vi "Name Value Metadata Interface.vi"(0 "Save Path":path, 7 "Input Tags Path":path) -> ()   [LabVIEW 2020]
uses:
  <vilib>/Utility/miscctls.llb/LVPointTypeDef.ctl
  Name Value Controls/Name Value Data Type Def.ctl
  <vilib>/Utility/file.llb/Read Delimited Spreadsheet (string).vi
panel:
  in  "Group Name Input":string
  in  "Tag Group 0":bool
  in  "Tag Group 6":bool
  in  "Tag Group 5":bool
  in  "Tag Group 4":bool
  in  "Tag Group 3":bool
  in  "Tag Group 2":bool
  in  "Tag Group 1":bool
  in  "Cancel":bool
  in  "Save":bool
  in  "Notes":string
  in  "Update Preset":bool
  in  "Save Preset":bool
  in  "Preset":u16(ring) items=["None", "Testing Two", "Testing"]
  in  "Clear All Tags":bool
  in  "Clear Tags":bool
  in  "Remove Group":bool
  in  "Add Group":bool
  in  "Metadata Tags":string[][](array[string])
  # "Name"
  # "Value"
  # "Value"
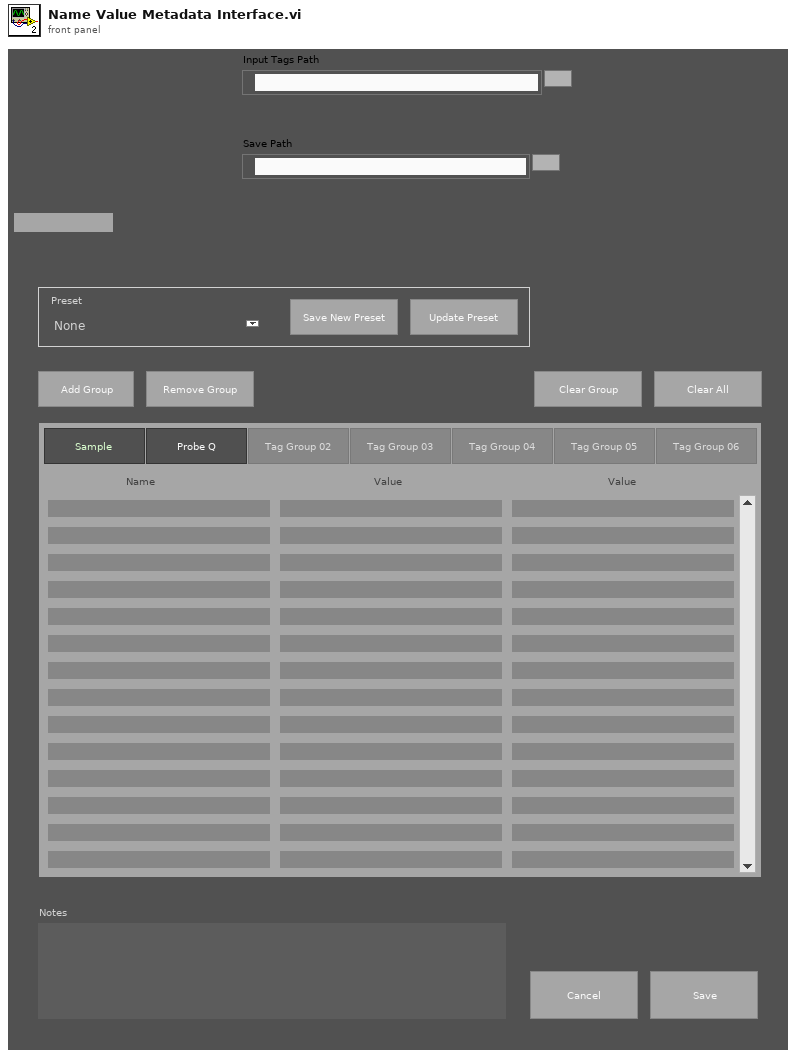
[diagram p1: front panel]
types:
  T1 = enum16{"Always On", "Always Off", "Off While Running"}
  T2 = typedef "LVPointTypeDef.ctl" = cluster{"Horizontal":i16, "Vertical":i16}
  T3 = enum8{"Enabled", "Disabled", "Disabled and Grayed Out"}
  T4 = typedef "Name Value Data Type Def.ctl" = cluster{"Sorted Tags":string[], "First Letters":string[], "Letter Indices":i32[]}
  T5 = typedef "LVBoundsTypeDef.ctl" = cluster{"Width":u32, "Height":u32}
  T6 = typedef "LVRectTypeDef.ctl" = cluster{"Left":i16, "Top":i16, "Right":i16, "Bottom":i16}
  T7 = enum32{"Invalid", "Standard", "Closed", "Hidden", "Minimized", "Maximized"}
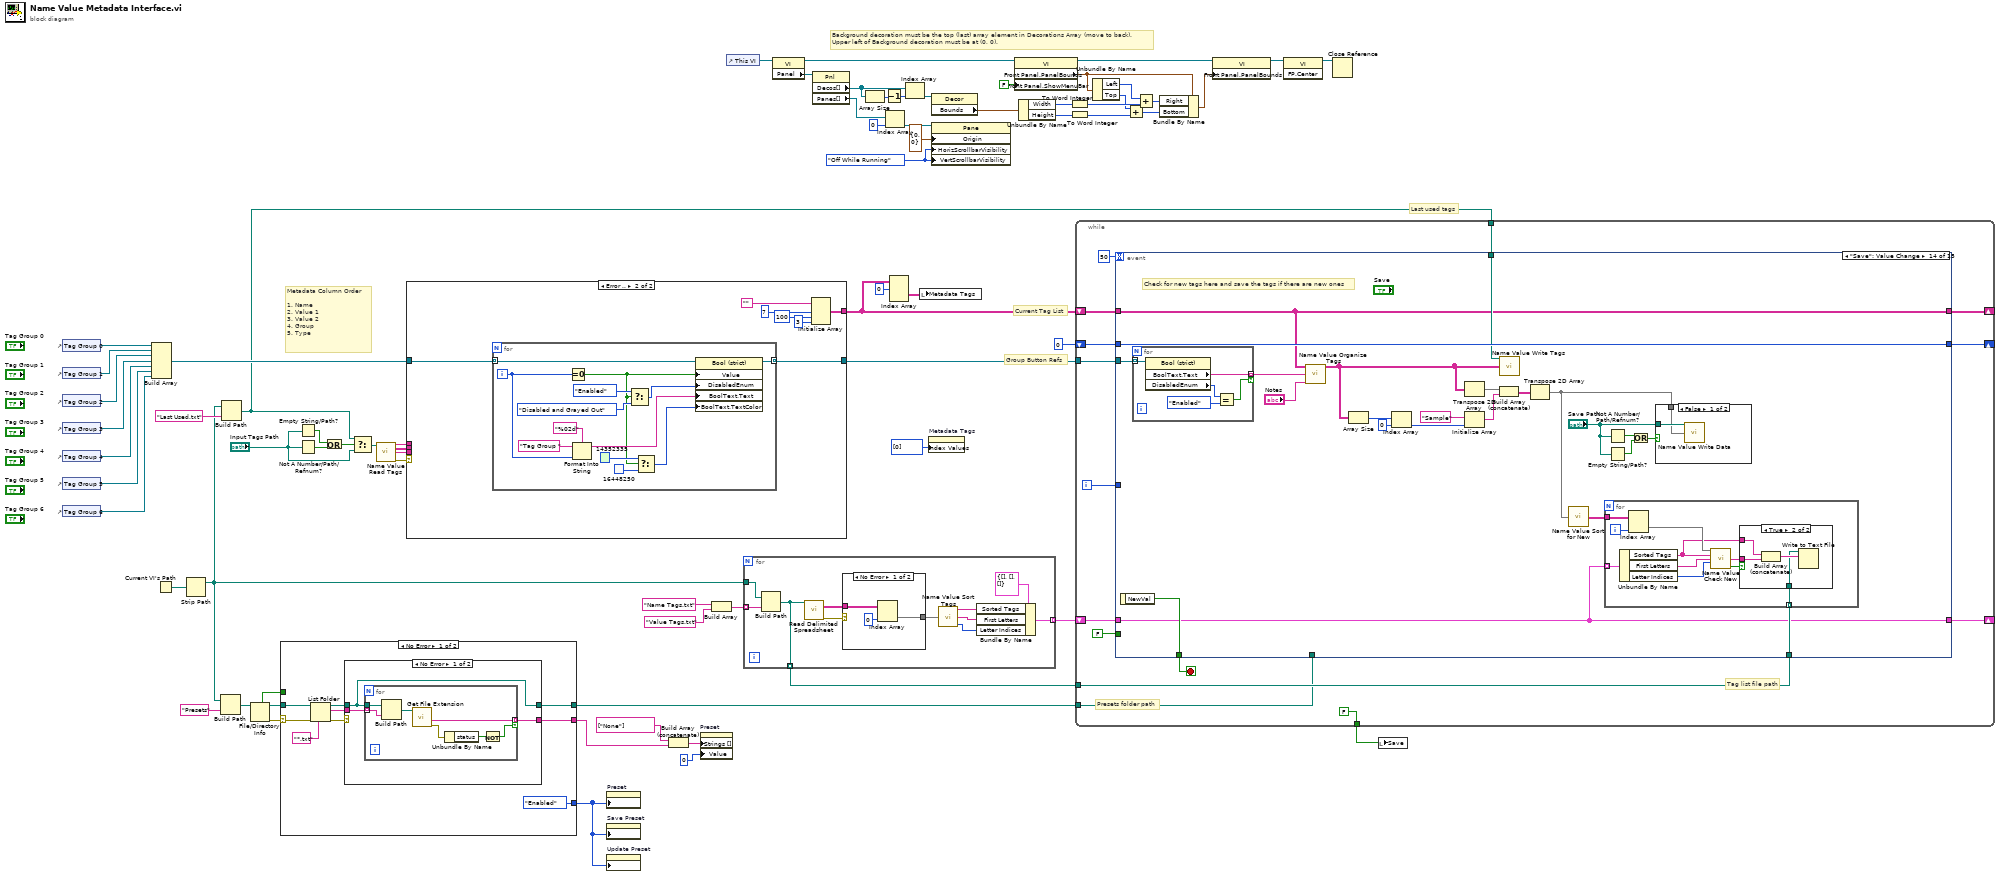
[diagram p0: block diagram]
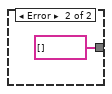
[diagram p2: hidden frame]
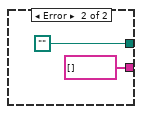
[diagram p3: hidden frame]
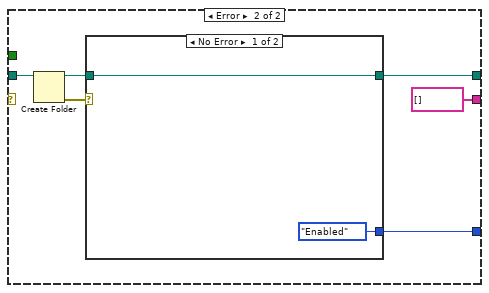
[diagram p4: hidden frame]
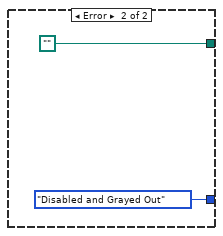
[diagram p5: hidden frame]
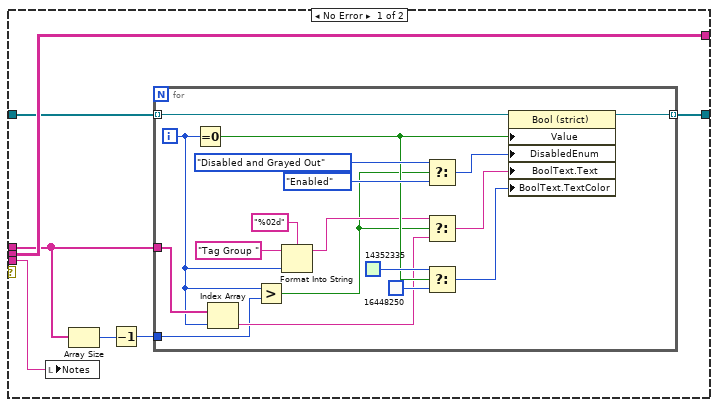
[diagram p6: hidden frame]
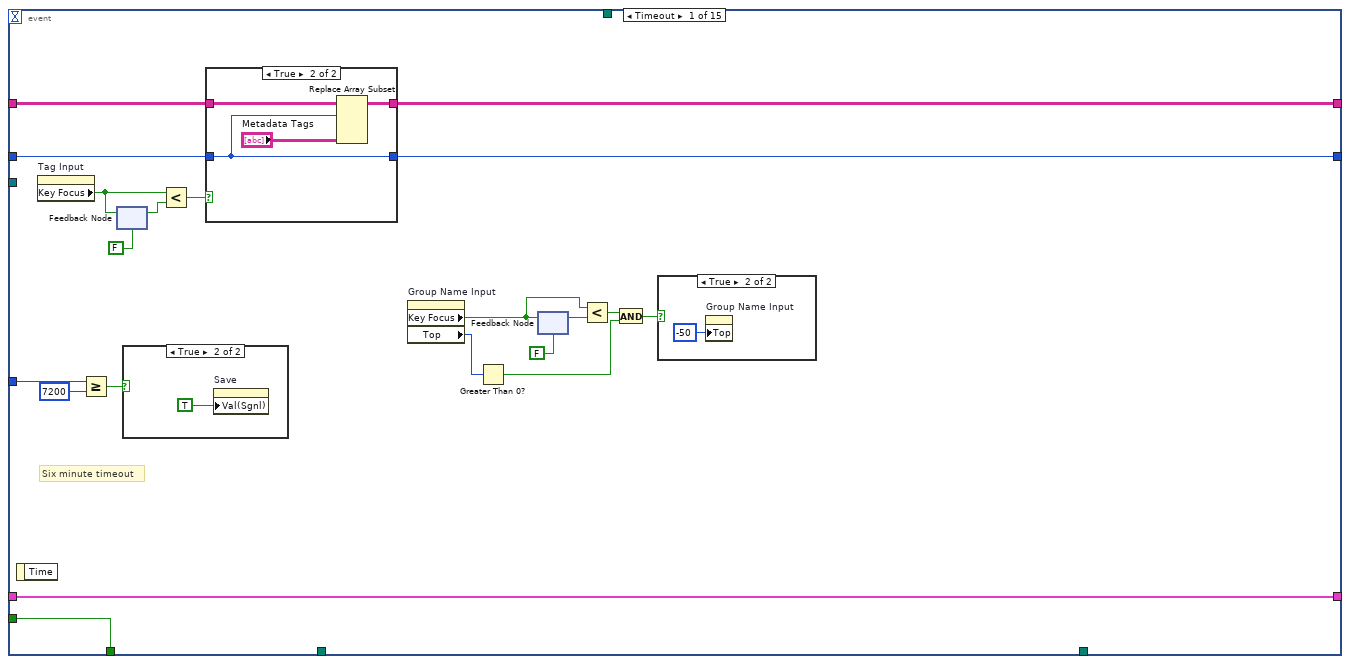
[diagram p7: hidden frame]
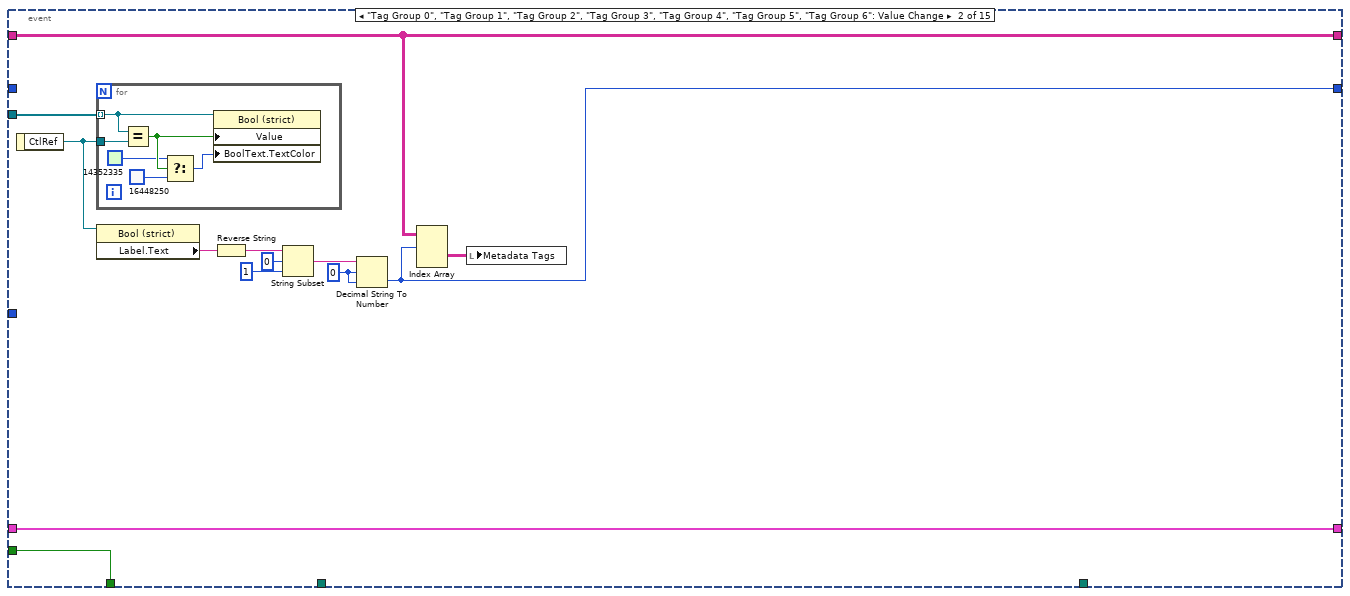
[diagram p11: hidden frame]
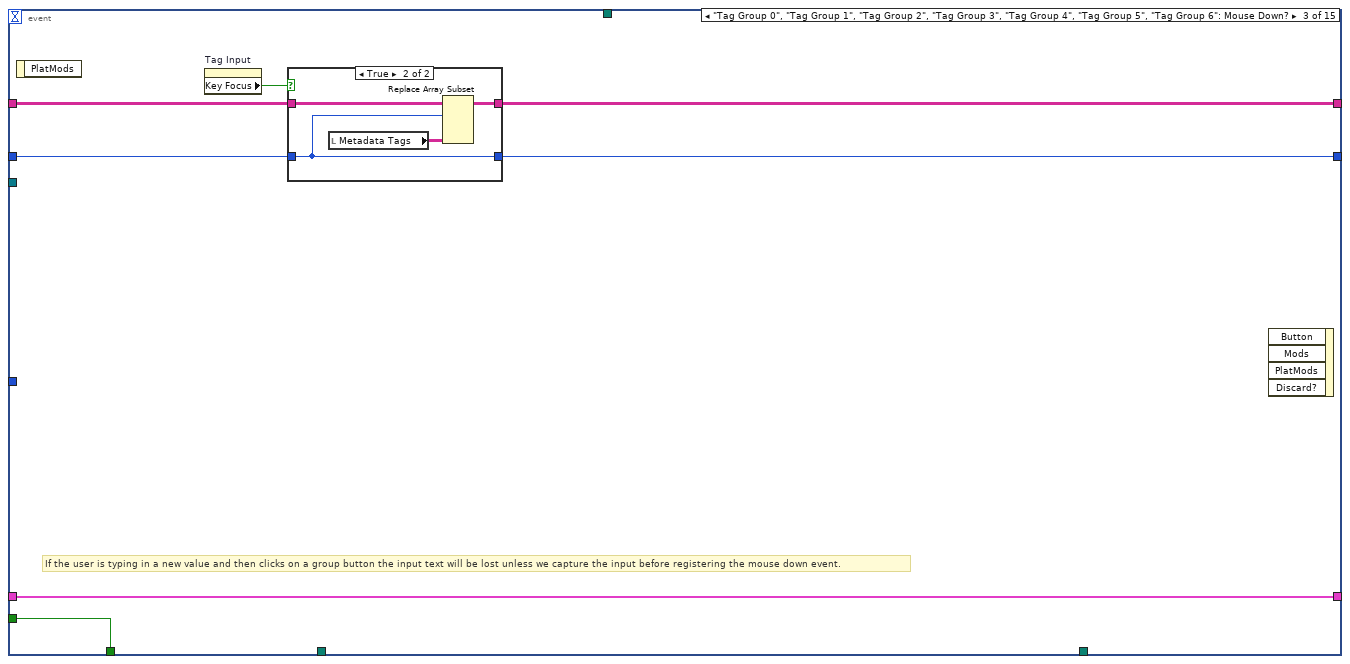
[diagram p12: hidden frame]
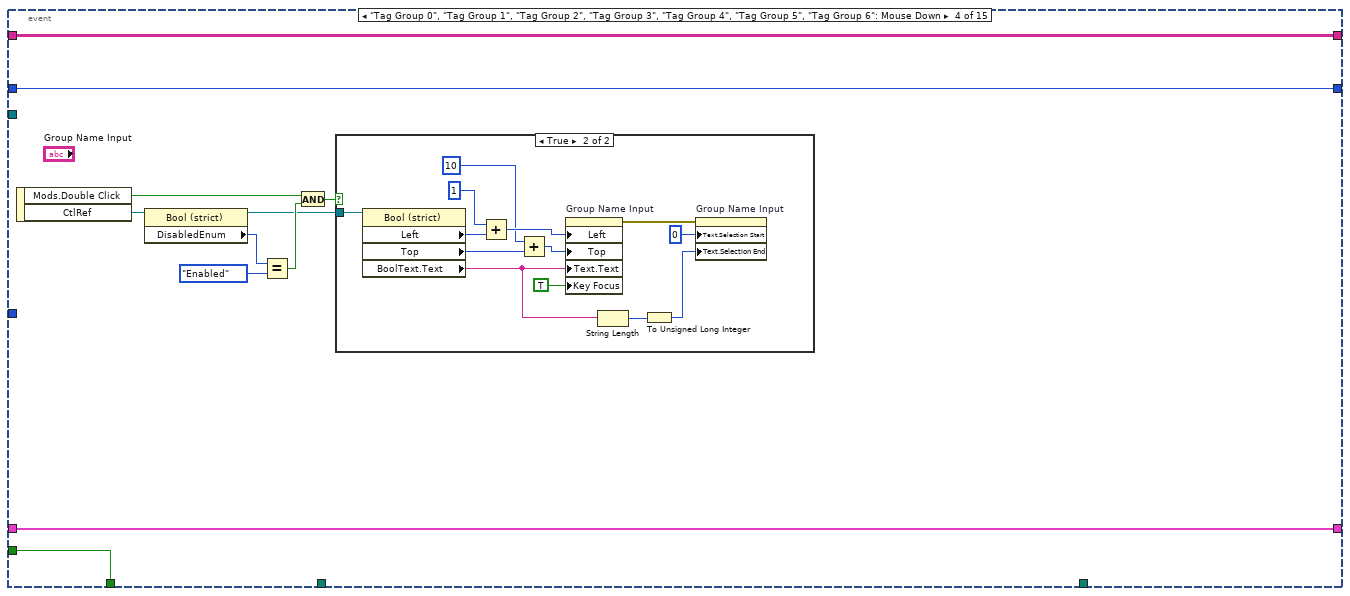
[diagram p14: hidden frame]
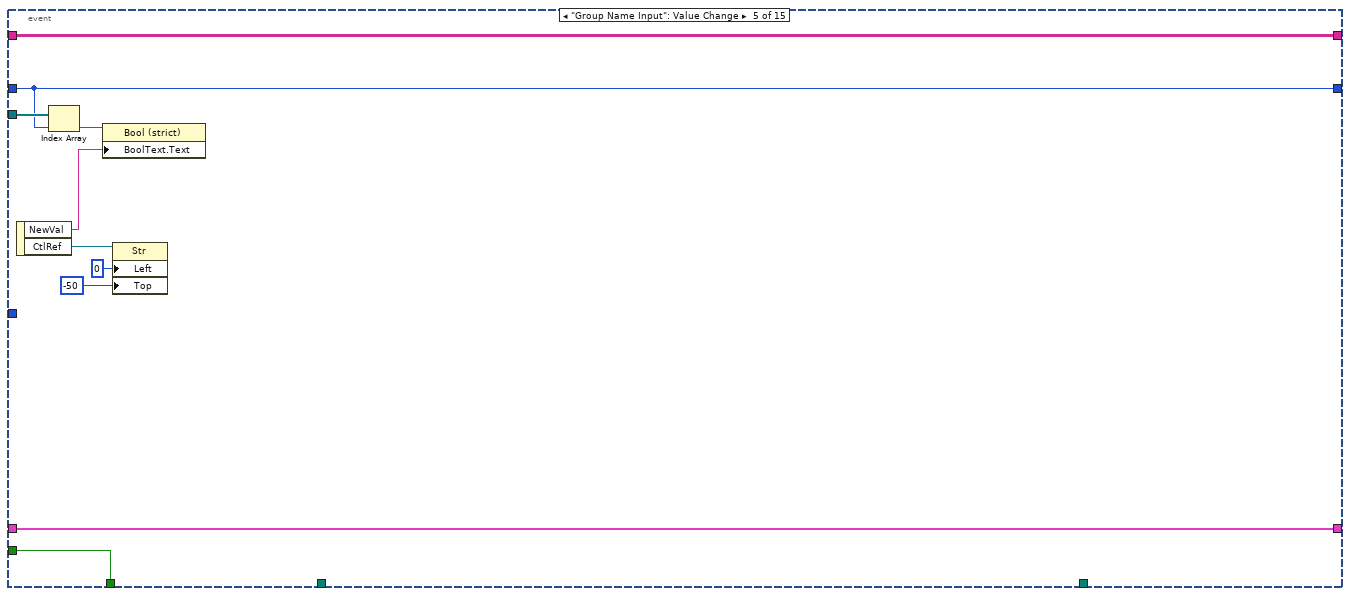
[diagram p16: hidden frame]
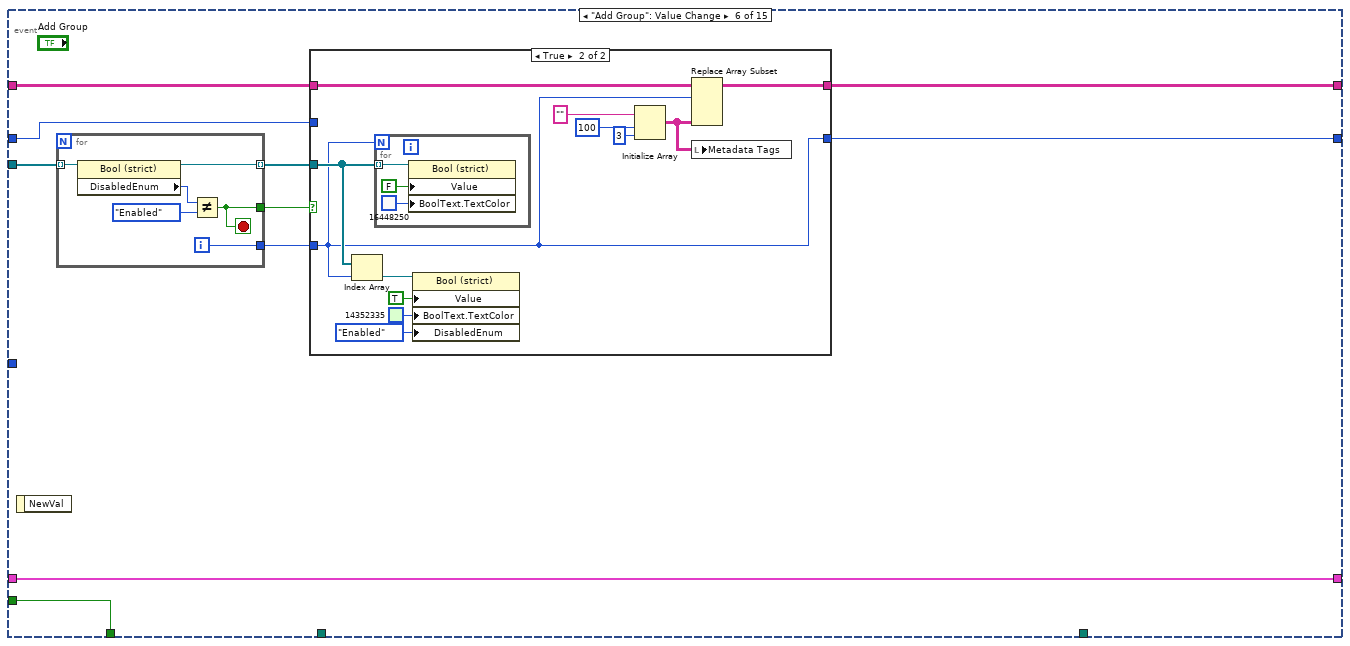
[diagram p17: hidden frame]
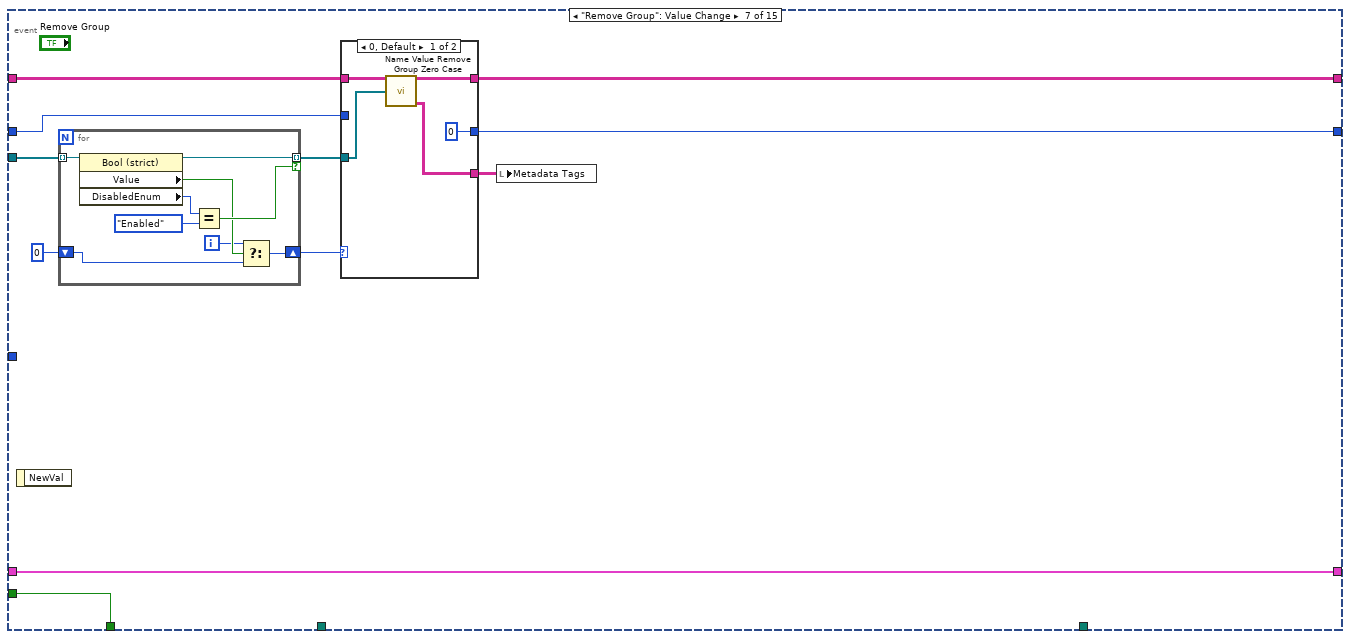
[diagram p19: hidden frame]
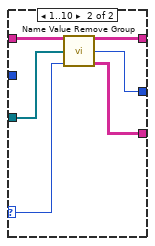
[diagram p20: hidden frame]
diagram:
  w62 = T1."Off While Running" ("Vertical Scrollbar Visibility")
  # "Last used tags"
  # "Group Button Refs"
  # "Metadata Column Order\n\n1. Name\n2. Value 1\n3. Value 2\n4. Group\n5. Type"
  # "Current Tag List"
  # "Background decoration must be the top (last) array element in Decorations Array (move to back).\nUpper left of Background decoration must be at (0, 0)."
  n1 = control-ref of="Tag Group 0"() -> (w46:refnum<vi>)
  n2 = control-ref of="Tag Group 1"() -> (w45:refnum<vi>)
  n3 = control-ref of="Tag Group 2"() -> (w44:refnum<vi>)
  n4 = control-ref of="Tag Group 3"() -> (w43:refnum<vi>)
  n5 = control-ref of="Tag Group 4"() -> (w42:refnum<vi>)
  n6 = control-ref of="Tag Group 5"() -> (w41:refnum<vi>)
  n7 = control-ref of="Tag Group 6"() -> (w40:refnum<vi>)
  n8 = Build Array(w46, w45, w44, w43, w42, w41, w40) -> (w38:refnum<vi>[])
  n9 = Current VI's Path() -> (path=w49:path)
  n10 = Strip Path(path=w49) -> (stripped path=w4:path)  [unwired: 1 out]
  n11 = Build Path(base path=w4, name or relative path="Presets") -> (appended path=w30:path)
  n12 = Build Path(base path=w4, name or relative path="Last Used.txt") -> (appended path=w15:path)
  n13 = File/Directory Info(path=w30) -> (path out=w27:path, directory=w28:bool, error out=w29:errorcluster)  [unwired: 1 in, 4 out]
  n14 = case shown="No Error" w29 {
    selector: w29 -> [w79 _]
    tunnel: w28 -> [_ _]
    tunnel: w27 -> [w80 w98]
    tunnel: [w73 w95] -> w22
    tunnel: [w75 string[] []] -> w24
    tunnel: [T3."Enabled" ("Disabled") w93] -> w21
    frame No Error {
      n15 = List Folder(path=w80, pattern="*.txt", error in=w79) -> (path out=w76:path, filenames=w77:string[], error out=w74:errorcluster)  [unwired: 1 in, 1 out]
      n16 = case shown="No Error" w74 {
        tunnel: w77 -> [w83 _]
        tunnel: w76 -> [w81 _]
        tunnel: [w82 string[] []] -> w75
        tunnel: [w81 path ""] -> w73
        frame No Error {
          n17 = for {
            tunnel: w83 -> [w89] mode=indexing
            tunnel: w81 -> [w90]
            tunnel: [w87] -> w82 mode=indexing if=w84
            n18 = Build Path(base path=w90, name or relative path=w89) -> (appended path=w88:path)
            n19 = call <vilib>:"Get File Extension.vi"("file"=w88) -> ("error out"=w86:errorcluster, "filename without extension"=w87:string)  [unwired: 6 in, 3 out]
            n20 = Unbundle By Name(w86) -> ("status"=w85:bool)
            n21 = Not(x=w85) -> (.not. x?=w84:bool)
          }
        }
        frame Error {
        }
      }
    }
    frame Error {
      n22 = Create Folder(path (use dialog)=w98) -> (created path=w96:path, error out=w97:errorcluster)  [unwired: 2 in, 1 out]
      n23 = case shown="No Error" w97 {
        tunnel: w96 -> [w100 _]
        tunnel: [w100 path ""] -> w95
        tunnel: [T3."Enabled" ("Disabled") T3."Disabled and Grayed Out" ("Disabled")] -> w93
        frame No Error {
        }
        frame Error {
        }
      }
    }
  }
  n24 = Empty String/Path?(string/path="Input Tags Path") -> (empty?=w19:bool)
  n25 = Not A Number/Path/Refnum?(number/path/refnum="Input Tags Path") -> (NaN/Path/Refnum?=w18:bool)
  n26 = Or(x=w19, y=w18) -> (x .or. y?=w17:bool)
  n27 = Select(t=w15, s=w17, f="Input Tags Path") -> (s? t:f=w20:path)
  n28 = call "Name Value Read Tags.vi"("Path"=w20) -> ("Group Names"=w34:string[], "Tags"=w33:string[][][], "Notes"=w32:string, "Error Out"=w35:errorcluster)  [unwired: 11 in]
  n29 = case shown="Error .." w35 {
    tunnel: w38 -> [w108 w134]
    tunnel: [w107 w133] -> w37
    tunnel: [w109 w130] -> w10
    tunnel: w34 -> [w106 _]
    tunnel: w33 -> [w109 _]
    tunnel: w32 -> [w103 _]
    frame No Error {
      n30 = local write "Notes"(w103) -> ()
      n31 = Array Size(array=w106) -> (size(s)=w105:i32)
      n32 = Decrement(x=w105) -> (x-1=w104:i32)
      n33 = for {
        tunnel: w108 -> [w127] mode=indexing
        tunnel: [w126] -> w107 mode=indexing
        tunnel: w106 -> [w114]
        tunnel: w104 -> [w110]
        i -> [w112]
        n34 = Equal To 0?(x=w112) -> (x = 0?=w117:bool)
        n35 = Index Array(array=w114, index=w112) -> (element=w113:string)
        n36 = Greater?(x=w112, y=w110) -> (0:w111:bool)
        n37 = Format Into String(format string="%02d", initial string="Tag Group ", w112) -> (resulting string=w116:string)  [unwired: 1 in, 1 out]
        n38 = Select(t=T3."Disabled and Grayed Out" ("Disabled"), s=w111, f=T3."Enabled" ("Disabled")) -> (s? t:f=w124:T3)
        n39 = Select(t=w116, s=w111, f=w113) -> (s? t:f=w115:string)
        n40 = Select(t=u32 14352335 ("Color Box"), s=w117, f=u32 16448250) -> (s? t:f=w118:u32)
        n41 = property class="Bool (strict)"(reference=w127, "Value"=w117, "DisabledEnum"=w124, "BoolText.Text"=w115, "BoolText.TextColor"=w118) -> (reference out=w126:refnum<vi>)  [unwired: 1 in, 1 out]
      }
    }
    frame Error {
      n42 = for {
        tunnel: w134 -> [w147] mode=indexing
        tunnel: [w146] -> w133 mode=indexing
        i -> [w140]
        n43 = Equal To 0?(x=w140) -> (x = 0?=w135:bool)
        n44 = Format Into String(format string="%02d", initial string="Tag Group ", w140) -> (resulting string=w139:string)  [unwired: 1 in, 1 out]
        n45 = Select(t=T3."Enabled" ("Disabled"), s=w135, f=T3."Disabled and Grayed Out" ("Disabled")) -> (s? t:f=w144:T3)
        n46 = Select(t=u32 14352335 ("Color Box"), s=w135, f=u32 16448250) -> (s? t:f=w136:u32)
        n47 = property class="Bool (strict)"(reference=w147, "Value"=w135, "DisabledEnum"=w144, "BoolText.Text"=w139, "BoolText.TextColor"=w136) -> (reference out=w146:refnum<vi>)  [unwired: 1 in, 1 out]
      }
      n48 = Initialize Array("", 7 ("dimension size"), 100 ("dimension size"), 3 ("dimension size")) -> (w130:string[][][])
    }
  }
  n49 = property on="Preset" class="Ring (strict)"("DisabledEnum"=w21) -> ()  [unwired: 2 in, 2 out]
  n50 = property on="Save Preset" class="Bool"("DisabledEnum"=w21) -> ()  [unwired: 2 in, 2 out]
  n51 = property on="Update Preset" class="Bool"("DisabledEnum"=w21) -> ()  [unwired: 2 in, 2 out]
  n52 = Build Array (concatenate)(string[] ["None"] ("Strings []"), w24) -> (w25:string[])
  n53 = property on="Preset" class="Ring (strict)"("Strings []"=w25, "Value"=u16 0) -> ()  [unwired: 2 in, 2 out]
  n54 = Build Array("Name Tags.txt", "Value Tags.txt") -> (w5:string[])
  n55 = control-ref of="This VI"() -> (w14:refnum<vi>)
  n56 = for {
    tunnel: [w151] -> w3 mode=indexing
    tunnel: w5 -> [w150] mode=indexing
    tunnel: w4 -> [w149]
    tunnel: [w148] -> w2 mode=indexing
    n57 = Build Path(base path=w149, name or relative path=w150) -> (appended path=w148:path)
    n58 = call-poly <vilib>:"Read Delimited Spreadsheet.vi"("file path (dialog if empty)"=w148) -> ("all rows"=w158:string[][], "error out"=w157:errorcluster)  [unwired: 9 in, 4 out]
    n59 = case shown="No Error" w157 {
      tunnel: w158 -> [w161 _]
      tunnel: [w159 string[] [] ("all rows")] -> w156
      frame No Error {
        n60 = Index Array(array=w161, index (col)=0 ("disabled index (col)")) -> (element=w159:string[])  [unwired: 1 in]
      }
      frame Error {
      }
    }
    n61 = call "Name Value Sort Tags.vi"("Tags"=w156) -> ("Sorted Tags"=w154:string[], "First Letters"=w153:string[], "Letter Indices"=w152:i32[])  [unwired: 12 in]
    n62 = Bundle By Name(cluster=T4 {"Sorted Tags"=[], "First Letters"=[], "Letter Indices"=[]} ("Tag Data"), "Sorted Tags"=w154, "First Letters"=w153, "Letter Indices"=w152) -> (w151:T4)
  }
  n63 = property class="VI"(reference=w14) -> (reference out=w63:refnum<vi>, "Panel"=w56:refnum<vi>)  [unwired: 1 in, 1 out]
  n64 = property class="Pnl"(reference=w56) -> ("Decos[]"=w48:refnum<vi>[], "Panes[]"=w59:refnum<vi>[])  [unwired: 1 in, 2 out]
  n65 = Array Size(array=w48) -> (size(s)=w55:i32)
  n66 = Decrement(x=w55) -> (x-1=w47:i32)
  n67 = Index Array(array=w59, index=0) -> (element=w58:refnum<vi>)
  n68 = Index Array(array=w10, index (dim 0)=0 ("index (page)")) -> (element=w8:string[][])  [unwired: 2 in]
  n69 = Index Array(array=w48, index=w47) -> (element=w61:refnum<vi>)
  n70 = local write "Metadata Tags"(w8) -> ()
  n71 = property on="Metadata Tags" class="Arr (strict)"("Index Values"=u32[] [0]) -> ()  [unwired: 2 in, 2 out]
  n72 = property class="Decor"(reference=w61) -> ("Bounds"=w64:T5)  [unwired: 1 in, 2 out]
  n73 = property class="Pane"(reference=w58, "Origin"=T2 {"Horizontal"=0, "Vertical"=0}, "HorizScrollbarVisibility"=w62, "VertScrollbarVisibility"=w62) -> ()  [unwired: 1 in, 2 out]
  n74 = property class="VI"(reference=w63, "Front Panel.ShowMenuBar"=FALSE ("Front Panel Window:Show Menu Bar")) -> (reference out=w65:refnum<vi>, "Front Panel.PanelBounds"=w66:T6)  [unwired: 1 in, 1 out]
  n75 = Unbundle By Name(w64) -> ("Width"=w69:u32, "Height"=w71:u32)
  n76 = To Word Integer(number=w69) -> (16bit integer=w70:i16)
  n77 = To Word Integer(number=w71) -> (16bit integer=w51:i16)
  n78 = while {
    tunnel: w37 -> [w175]
    shift-right: [w168] -> _
    shift-left: w10 -> [w174]
    shift-right: [w172] -> _
    shift-left: 0 -> [w173]
    tunnel: w2 -> [w170]
    tunnel: w15 -> [w169]
    tunnel: w22 -> [w167]
    shift-right: [w164] -> _
    shift-left: w3 -> [w165]
    tunnel: [FALSE] -> w1
    i -> [w166]
    stop <- w176 stop-if-true
    # "Presets folder path"
    # "Tag list file path"
    n79 = event shown="[13] \"Save\": Value Change" {
      selector: _ -> [_ _ _ _ _ _ _ _ _ _ _ _ _ _ _]
      dyn-events: _ -> [_ _ _ _ _ _ _ _ _ _ _ _ _ _ _]
      timeout: 50 -> [_ _ _ _ _ _ _ _ _ _ _ _ _ _ _]
      tunnel: FALSE -> [w197 w218 w231 w248 w271 w281 w315 w363 w389 w399 w419 w465 w491 _ _]
      tunnel: [w197 w218 w231 w248 w271 w281 w315 w363 w389 w399 w419 w465 w491 w532 TRUE ("NewVal")] -> w176
      tunnel: w175 -> [_ w217 _ _ w266 w273 w314 _ _ _ w409 w463 w489 w530 _]
      tunnel: [w190 w208 w229 w247 w270 w275 w310 w351 w385 w392 w402 w450 w480 w523 w556] -> w168
      tunnel: w174 -> [w192 w208 w230 w247 w270 w276 w311 w351 w386 _ w405 w450 w480 w523 w556]
      tunnel: w173 -> [w191 _ w228 w246 w265 w279 w309 w352 w382 w398 w404 w464 w484 w531 w555]
      tunnel: [w189 w207 w227 w246 w265 w277 w308 w352 w382 w398 w403 w464 w483 w531 w555] -> w172
      tunnel: w170 -> [_ _ _ _ _ _ _ _ _ _ _ _ _ w513 _]
      tunnel: w169 -> [_ _ _ _ _ _ _ _ _ _ _ _ _ w529 _]
      tunnel: w167 -> [_ _ _ _ _ _ _ _ _ _ w411 w458 w487 _ _]
      tunnel: w166 -> [w181 _ _ _ _ _ _ _ _ _ _ _ _ _ _]
      tunnel: w165 -> [w178 w209 w225 w238 w262 w272 w305 w344 w384 w393 w401 w452 w481 w512 w554]
      tunnel: [w178 w209 w225 w238 w262 w272 w305 w344 w384 w393 w401 w452 w481 w512 w554] -> w164
      event Timeout {
        # "Six minute timeout"
        n80 = event-data() -> ()  [unwired: 1 in, 1 out]
        n81 = property on="Tag Input" class="Str"() -> ("Key Focus"=w195:bool)  [unwired: 2 in, 2 out]
        n82 = Greater Or Equal?(x=w181, y=7200) -> (x >= y?=w179:bool)
        n83 = feedback-in #1(w195) -> ()
        n84 = feedback #1(FALSE ("Key Focus")) -> (w196:bool)
        n85 = case shown="True" w179 {
          frame False {
          }
          frame True {
            n86 = property on="Save" class="Bool (strict)"("Val(Sgnl)"=TRUE) -> ()  [unwired: 2 in, 2 out]
          }
        }
        n87 = Less?(x=w195, y=w196) -> (x < y?=w193:bool)
        n88 = case shown="True" w193 {
          tunnel: w192 -> [w201 w205]
          tunnel: w191 -> [w200 w202]
          tunnel: [w201 w204] -> w190
          tunnel: [w200 w202] -> w189
          frame False {
          }
          frame True {
            n89 = Replace Array Subset(array=w205, new element="Metadata Tags", index (dim 0)=w202) -> (w204:string[][][])  [unwired: 2 in]
          }
        }
        n90 = property on="Group Name Input" class="Str"() -> ("Key Focus"=w186:bool, "Top"=w185:i32)  [unwired: 2 in, 2 out]
        n91 = Greater Than 0?(x=w185) -> (x > 0?=w183:bool)
        n92 = feedback #2(FALSE ("Key Focus")) -> (w188:bool)
        n93 = feedback-in #2(w186) -> ()
        n94 = Less?(x=w186, y=w188) -> (x < y?=w184:bool)
        n95 = And(x=w184, y=w183) -> (x .and. y?=w182:bool)
        n96 = case shown="True" w182 {
          frame False {
          }
          frame True {
            n97 = property on="Group Name Input" class="Str"("Top"=-50 ("Position:Top")) -> ()  [unwired: 2 in, 2 out]
          }
        }
      }
      event "Tag Group 0", "Tag Group 1", "Tag Group 2", "Tag Group 3", "Tag Group 4", "Tag Group 5", "Tag Group 6": Value Change {
        w210 = 0 ("offset")
        n98 = event-data() -> ("CtlRef"=w216:refnum<vi>)  [unwired: 1 in]
        n99 = for {
          tunnel: w217 -> [w223] mode=indexing
          tunnel: w216 -> [w224]
          n100 = Equal?(x=w223, y=w224) -> (x = y?=w222:bool)
          n101 = Select(t=u32 14352335 ("Color Box"), s=w222, f=u32 16448250) -> (s? t:f=w220:u32)
          n102 = property class="Bool (strict)"(reference=w223, "Value"=w222, "BoolText.TextColor"=w220) -> ()  [unwired: 1 in, 2 out]
        }
        n103 = property class="Bool (strict)"(reference=w216) -> ("Label.Text"=w215:string)  [unwired: 1 in, 2 out]
        n104 = Reverse String(1:w215) -> (0:w214:string)
        n105 = String Subset(string=w214, offset (0)=0, length (rest)=1 ("length (rest)")) -> (substring=w211:string)
        n106 = Decimal String To Number(string=w211, offset=w210, default (0L)=w210) -> (number=w207:i32)  [unwired: 1 out]
        n107 = Index Array(array=w208, index (dim 0)=w207) -> (element=w206:string[][])  [unwired: 2 in]
        n108 = local write "Metadata Tags"(w206) -> ()
      }
      event "Tag Group 0", "Tag Group 1", "Tag Group 2", "Tag Group 3", "Tag Group 4", "Tag Group 5", "Tag Group 6": Mouse Down? {
        # "If the user is typing in a new value and then clicks on a group button the input text will be lost unless we capture the input before registering the mouse down event."
        n109 = event-data() -> ()  [unwired: 1 in, 1 out]
        n110 = property on="Tag Input" class="Str"() -> ("Key Focus"=w226:bool)  [unwired: 2 in, 2 out]
        n111 = case shown="True" w226 {
          tunnel: w230 -> [w233 w237]
          tunnel: w228 -> [w232 w235]
          tunnel: [w233 w236] -> w229
          tunnel: [w232 w235] -> w227
          frame False {
          }
          frame True {
            n112 = local read "Metadata Tags"() -> (w234:string[][])
            n113 = Replace Array Subset(array=w237, new element=w234, index (dim 0)=w235) -> (w236:string[][][])  [unwired: 2 in]
          }
        }
        n114 = event-data() -> ()  [unwired: 5 in, 1 out]
      }
      event "Tag Group 0", "Tag Group 1", "Tag Group 2", "Tag Group 3", "Tag Group 4", "Tag Group 5", "Tag Group 6": Mouse Down {
        n115 = event-data() -> ("Mods.Double Click"=w242:bool, "CtlRef"=w245:refnum<vi>)  [unwired: 1 in]
        n116 = property class="Bool (strict)"(reference=w245) -> (reference out=w240:refnum<vi>, "DisabledEnum"=w244:T3)  [unwired: 1 in, 1 out]
        n117 = Equal?(x=w244, y=T3."Enabled") -> (x = y?=w241:bool)
        n118 = And(x=w242, y=w241) -> (x .and. y?=w239:bool)
        n119 = case shown="True" w239 {
          tunnel: w240 -> [_ w261]
          frame False {
          }
          frame True {
            n120 = property class="Bool (strict)"(reference=w261) -> ("Left"=w254:i32, "Top"=w251:i32, "BoolText.Text"=w258:string)  [unwired: 1 in, 2 out]
            n121 = Add(x=1 ("Left"), y=w254) -> (x+y=w252:i32)
            n122 = Add(x=10 ("Top"), y=w251) -> (x+y=w250:i32)
            n123 = property on="Group Name Input" class="Str"("Left"=w252, "Top"=w250, "Text.Text"=w258, "Key Focus"=TRUE) -> (error out=w260:errorcluster)  [unwired: 2 in, 1 out]
            n124 = String Length(string=w258) -> (length=w257:i32)
            n125 = To Unsigned Long Integer(number=w257) -> (unsigned 32bit integer=w256:u32)
            n126 = property on="Group Name Input" class="Str"(error in=w260, "Text.Selection Start"=u32 0 ("Text.Selection:Start"), "Text.Selection End"=w256) -> ()  [unwired: 1 in, 2 out]
          }
        }
      }
      event "Group Name Input": Value Change {
        n127 = event-data() -> ("NewVal"=w263:string, "CtlRef"=w269:refnum<vi>)  [unwired: 1 in]
        n128 = Index Array(array=w266, index=w265) -> (element=w264:refnum<vi>)
        n129 = property class="Bool (strict)"(reference=w264, "BoolText.Text"=w263) -> ()  [unwired: 1 in, 2 out]
        n130 = property class="Str"(reference=w269, "Left"=0 ("Position:Left"), "Top"=-50 ("Position:Top")) -> ()  [unwired: 1 in, 2 out]
      }
      event "Add Group": Value Change {
        n131 = event-data() -> ()  [unwired: 1 in, 1 out]
        n132 = for {
          tunnel: w273 -> [w303] mode=indexing
          tunnel: [w302] -> w274 mode=indexing
          tunnel: [w301] -> w280
          tunnel: [w300] -> w278
          i -> [w300]
          stop <- w301 stop-if-true
          n133 = property class="Bool (strict)"(reference=w303) -> (reference out=w302:refnum<vi>, "DisabledEnum"=w299:T3)  [unwired: 1 in, 1 out]
          n134 = Not Equal?(x=w299, y=T3."Enabled") -> (x != y?=w301:bool)
        }
        n135 = case shown="True" w280 {
          tunnel: w279 -> [w283 _]
          tunnel: w278 -> [_ w286]
          tunnel: [w283 w286] -> w277
          tunnel: w276 -> [w282 w293]
          tunnel: [w282 w292] -> w275
          tunnel: w274 -> [_ w291]
          frame False {
          }
          frame True {
            n136 = Index Array(array=w291, index=w286) -> (element=w290:refnum<vi>)
            n137 = for {
              N: w286 -> [_]
              tunnel: w291 -> [w296] mode=indexing
              n138 = property class="Bool (strict)"(reference=w296, "Value"=FALSE, "BoolText.TextColor"=u32 16448250) -> ()  [unwired: 1 in, 2 out]
            }
            n139 = property class="Bool (strict)"(reference=w290, "Value"=TRUE, "BoolText.TextColor"=u32 14352335 ("Color Box"), "DisabledEnum"=T3."Enabled" ("Disabled")) -> ()  [unwired: 1 in, 2 out]
            n140 = Initialize Array("", 100 ("dimension size"), 3 ("dimension size")) -> (w284:string[][])
            n141 = Replace Array Subset(array=w293, new element=w284, index (dim 0)=w286) -> (w292:string[][][])  [unwired: 2 in]
            n142 = local write "Metadata Tags"(w284) -> ()
          }
        }
      }
      event "Remove Group": Value Change {
        n143 = event-data() -> ()  [unwired: 1 in, 1 out]
        n144 = for {
          tunnel: w314 -> [w335] mode=indexing
          tunnel: [w332] -> w312 mode=indexing if=w331
          shift-right: [w328] -> w307
          shift-left: 0 -> [w329]
          i -> [w327]
          n145 = property class="Bool (strict)"(reference=w335) -> (reference out=w332:refnum<vi>, "Value"=w330:bool, "DisabledEnum"=w334:T3)  [unwired: 1 in, 1 out]
          n146 = Equal?(x=w334, y=T3."Enabled") -> (x = y?=w331:bool)
          n147 = Select(t=w327, s=w330, f=w329) -> (s? t:f=w328:i32)
        }
        n148 = case shown="0, Default" w307 {
          selector: w307 -> [_ w325]
          tunnel: w312 -> [w317 w324]
          tunnel: w311 -> [w320 w326]
          tunnel: [w319 w322] -> w310
          tunnel: w309 -> [_ _]
          tunnel: [0 ("Update Index") w323] -> w308
          tunnel: [w318 w321] -> w306
          frame 0, Default {
            n149 = call "Name Value Remove Group Zero Case.vi"("Tags Array"=w320, "Boolean Refs Array"=w317) -> ("Updated Tag Array"=w319:string[][][], "Current Tags"=w318:string[][])  [unwired: 12 in]
          }
          frame 1..10 {
            n150 = call "Name Value Remove Group.vi"("Tags Array"=w326, "Boolean Refs Array"=w324, "Group Index"=w325) -> ("Updated Tag Array"=w322:string[][][], "Update Index"=w323:i32, "Current Tags"=w321:string[][])  [unwired: 10 in]
          }
        }
        n151 = local write "Metadata Tags"(w306) -> ()
      }
      event "Metadata Tags": Value Change {
        w357 = refnum<vi> refnum  # String
        # "Check if input is from column 1 (names) or other columns (values)."
        n152 = event-data() -> ("CtlRef"=w361:refnum<vi>, "OldVal"=w347:string[][], "NewVal"=w346:string[][])  [unwired: 1 in]
        n153 = Not Equal?(x=w347, y=w346) -> (x != y?=w349:bool[][])
        n154 = Transpose 2D Array(2D array=w349) -> (transposed array=w348:bool[][])
        n155 = for {
          tunnel: w348 -> [w366] mode=indexing
          tunnel: [w364] -> w345
          i -> [w364]
          stop <- w365 stop-if-true
          n156 = Or Array Elements(Boolean array=w366) -> (logical OR=w365:bool)
        }
        n157 = Greater Than 0?(x=w345) -> (x > 0?=w339:bool)
        n158 = Select(t=1, s=w339, f=0) -> (s? t:f=w336:i32)
        n159 = property class="Arr (strict)"(reference=w361) -> ("Array Element"=w358:refnum<vi>, "Array Element.Value"=w354:variant)  [unwired: 1 in, 2 out]
        n160 = Index Array(array=w344, index=w336) -> (element=w343:T4)
        n161 = Unbundle By Name(w343) -> ("Sorted Tags"=w342:string[], "First Letters"=w341:string[], "Letter Indices"=w340:i32[])
        n162 = Variant To Data(type="", Variant=w354) -> (data=w356:string)  [unwired: 1 in, 1 out]
        n163 = To More Specific Class(target class=w357, reference=w358) -> (specific class reference=w350:refnum<vi>)  [unwired: 1 in, 1 out]
        n164 = call "Popup Menu Get State.vi"() -> ("FP State"=w360:T7, "Error Out"=w359:errorcluster)  [unwired: 14 in]
        n165 = call "Name Value AutoComplete Items.vi"("Input String"=w356, "Match Limit"=10, "Sorted Tags"=w342, "First Letters"=w341, "Letter Indicies"=w340) -> ("AutoComplete"=w353:string[])  [unwired: 10 in]
        n166 = case shown="\"Closed\"" w360 {
          tunnel: w350 -> [_ w373 _]
          tunnel: w359 -> [_ w369 w377]
          tunnel: w353 -> [_ w368 w374]
          frame Default {
          }
          frame "Closed" {
            n167 = control-ref of="This VI"() -> (w372:refnum<vi>)
            n168 = call "Popup Menu Get XY.vi"("Vert Adj"=i16 33, "VI Ref"=w372, "Str Ctrl Ref"=w373, "Errror In"=w369) -> ("Screen Coordinates"=w371:T2, "Error Out"=w370:errorcluster)  [unwired: 10 in]
            n169 = call "Popup Menu Start.vi"("VI Ref"=w372, "Str Ctrl Ref"=w373, "Initial Menu Options"=w368, "Error In"=w370, "XY Position"=w371) -> ()  [unwired: 10 in, 1 out]
          }
          frame "Standard" {
            n170 = Array Size(array=w374) -> (size(s)=w376:i32)
            n171 = Greater Than 0?(x=w376) -> (x > 0?=w375:bool)
            n172 = case shown="False" w375 {
              tunnel: w377 -> [w378 w380]
              tunnel: w374 -> [_ w379]
              frame False {
                n173 = call "Popup Menu Close.vi"("Error In"=w378) -> ()  [unwired: 14 in, 1 out]
              }
              frame True {
                n174 = call "Popup Menu Update Items.vi"("Menu Items"=w379, "Error In"=w380) -> ()  [unwired: 13 in, 1 out]
              }
            }
          }
        }
      }
      event "Clear Tags": Value Change {
        n175 = event-data() -> ()  [unwired: 1 in, 6 out]
        n176 = Initialize Array("", 100 ("dimension size"), 3 ("dimension size")) -> (w381:string[][])
        n177 = Replace Array Subset(array=w386, new element=w381, index (dim 0)=w382) -> (w385:string[][][])  [unwired: 2 in]
        n178 = local write "Metadata Tags"(w381) -> ()
      }
      event "Clear All Tags": Value Change {
        n179 = event-data() -> ()  [unwired: 1 in, 6 out]
        n180 = Initialize Array("", 7 ("dimension size"), 100 ("dimension size"), 3 ("dimension size")) -> (w392:string[][][])
        n181 = Index Array(array=w392, index (dim 0)=0 ("index (page)")) -> (element=w390:string[][])  [unwired: 2 in]
        n182 = local write "Metadata Tags"(w390) -> ()
      }
      event "Preset": Value Change {
        n183 = event-data() -> ("CtlRef"=w418:refnum<vi>, "NewVal"=w416:u16)  [unwired: 1 in]
        n184 = property class="Ring (strict)"(reference=w418) -> ("Strings []"=w417:string[])  [unwired: 1 in, 2 out]
        n185 = To Long Integer(number=w416) -> (32bit integer=w415:i32)
        n186 = Index Array(array=w417, index=w415) -> (element=w414:string)
        n187 = Concatenate Strings(w414, ".txt" ("string")) -> (w412:string)
        n188 = Build Path(base path=w411, name or relative path=w412) -> (appended path=w410:path)
        n189 = call "Name Value Read Tags.vi"("Path"=w410) -> ("Group Names"=w408:string[], "Tags"=w407:string[][][], "Notes"=w400:string, "Error Out"=w406:errorcluster)  [unwired: 11 in]
        n190 = case shown="No Error" w406 {
          tunnel: w409 -> [w428 _]
          tunnel: [w422 w447] -> w402
          tunnel: w408 -> [w427 _]
          tunnel: w407 -> [w422 _]
          tunnel: w400 -> [w424 _]
          tunnel: w405 -> [_ w447]
          tunnel: w404 -> [_ w446]
          tunnel: [0 w446] -> w403
          frame No Error {
            n191 = local write "Notes"(w424) -> ()
            n192 = Index Array(array=w422, index (dim 0)=0 ("index (page)")) -> (element=w420:string[][])  [unwired: 2 in]
            n193 = Array Size(array=w427) -> (size(s)=w426:i32)
            n194 = Decrement(x=w426) -> (x-1=w425:i32)
            n195 = local write "Metadata Tags"(w420) -> ()
            n196 = for {
              tunnel: w428 -> [w445] mode=indexing
              tunnel: w427 -> [w433]
              tunnel: w425 -> [w429]
              i -> [w431]
              n197 = Equal To 0?(x=w431) -> (x = 0?=w436:bool)
              n198 = Index Array(array=w433, index=w431) -> (element=w432:string)
              n199 = Greater?(x=w431, y=w429) -> (0:w430:bool)
              n200 = Format Into String(format string="%02d", initial string="Tag Group ", w431) -> (resulting string=w435:string)  [unwired: 1 in, 1 out]
              n201 = Select(t=T3."Disabled and Grayed Out" ("Disabled"), s=w430, f=T3."Enabled" ("Disabled")) -> (s? t:f=w443:T3)
              n202 = Select(t=w435, s=w430, f=w432) -> (s? t:f=w434:string)
              n203 = Select(t=u32 14352335 ("Color Box"), s=w436, f=u32 16448250) -> (s? t:f=w437:u32)
              n204 = property class="Bool (strict)"(reference=w445, "Value"=w436, "DisabledEnum"=w443, "BoolText.Text"=w434, "BoolText.TextColor"=w437) -> ()  [unwired: 1 in, 2 out]
            }
          }
          frame Error {
          }
        }
      }
      event "Save Preset": Value Change {
        n205 = event-data() -> ()  [unwired: 1 in, 1 out]
        n206 = for {
          tunnel: w463 -> [w478] mode=indexing
          tunnel: [w476] -> w451 mode=indexing if=w475
          n207 = property class="Bool (strict)"(reference=w478) -> ("BoolText.Text"=w476:string, "DisabledEnum"=w477:T3)  [unwired: 1 in, 2 out]
          n208 = Equal?(x=w477, y=T3."Enabled") -> (x = y?=w475:bool)
        }
        n209 = call "Name Value Get User Input.vi"("Dialog Message"="Preset Name") -> ("User Input"=w455:string, "Canceled?"=w457:bool)  [unwired: 13 in]
        n210 = control-ref of="Preset"() -> (w462:refnum<vi>)
        n211 = local read "Notes"() -> (w449:string)
        n212 = Concatenate Strings(w455, ".txt" ("string")) -> (w459:string)
        n213 = property class="Ring (strict)"(reference=w462) -> (reference out=w453:refnum<vi>, "Strings []"=w454:string[])  [unwired: 1 in, 1 out]
        n214 = call "Name Value Organize Tags.vi"("Name Values"=w450, "Group Names"=w451, "Notes"=w449) -> ("Name Value Group"=w448:string[][])  [unwired: 12 in]
        n215 = Build Path(base path=w458, name or relative path=w459) -> (appended path=w456:path)
        n216 = case shown="False" w457 {
          tunnel: w448 -> [w474 _]
          tunnel: w456 -> [w473 _]
          tunnel: w455 -> [w471 _]
          tunnel: w454 -> [w472 _]
          tunnel: w453 -> [w469 _]
          frame False {
            n217 = call "Name Value Write Tags.vi"("File Path"=w473, "Tags Group Array"=w474) -> ()  [unwired: 13 in, 1 out]
            n218 = Build Array (concatenate)(w472, w471) -> (w466:string[])
            n219 = Array Size(array=w466) -> (size(s)=w470:i32)
            n220 = Decrement(x=w470) -> (x-1=w468:i32)
            n221 = To Unsigned Word Integer(number=w468) -> (unsigned 16bit integer=w467:u16)
            n222 = property class="Ring (strict)"(reference=w469, "Strings []"=w466, "Value"=w467) -> ()  [unwired: 1 in, 2 out]
          }
          frame True {
          }
        }
      }
      event "Update Preset": Value Change {
        n223 = event-data() -> ()  [unwired: 1 in, 1 out]
        n224 = for {
          tunnel: w489 -> [w508] mode=indexing
          tunnel: [w506] -> w490 mode=indexing if=w505
          n225 = property class="Bool (strict)"(reference=w508) -> ("BoolText.Text"=w506:string, "DisabledEnum"=w507:T3)  [unwired: 1 in, 2 out]
          n226 = Equal?(x=w507, y=T3."Enabled") -> (x = y?=w505:bool)
        }
        n227 = control-ref of="Preset"() -> (w488:refnum<vi>)
        n228 = property class="Ring (strict)"(reference=w488) -> ("Strings []"=w486:string[], "Value"=w485:u16)  [unwired: 1 in, 2 out]
        n229 = To Long Integer(number=w485) -> (32bit integer=w482:i32)
        n230 = case shown="Default" w482 {
          selector: w482 -> [_ w497]
          tunnel: w490 -> [_ w496]
          tunnel: w487 -> [_ w502]
          tunnel: w486 -> [_ w500]
          tunnel: w484 -> [w492 w498]
          tunnel: [w492 w498] -> w483
          tunnel: w480 -> [_ w495]
          frame 0 {
          }
          frame Default {
            n231 = local read "Notes"() -> (w494:string)
            n232 = Index Array(array=w500, index=w497) -> (element=w499:string)
            n233 = call "Name Value Organize Tags.vi"("Name Values"=w495, "Group Names"=w496, "Notes"=w494) -> ("Name Value Group"=w493:string[][])  [unwired: 12 in]
            n234 = Concatenate Strings(w499, ".txt" ("string")) -> (w503:string)
            n235 = Build Path(base path=w502, name or relative path=w503) -> (appended path=w501:path)
            n236 = call "Name Value Write Tags.vi"("File Path"=w501, "Tags Group Array"=w493) -> ()  [unwired: 13 in, 1 out]
          }
        }
      }
      event "Save": Value Change {
        # "Check for new tags here and save the tags if there are new ones"
        n237 = event-data() -> ("NewVal"=w532:bool)  [unwired: 1 in]
        n238 = for {
          tunnel: w530 -> [w552] mode=indexing
          tunnel: [w550] -> w524 mode=indexing if=w549
          n239 = property class="Bool (strict)"(reference=w552) -> ("BoolText.Text"=w550:string, "DisabledEnum"=w551:T3)  [unwired: 1 in, 2 out]
          n240 = Equal?(x=w551, y=T3."Enabled") -> (x = y?=w549:bool)
        }
        n241 = call "Name Value Organize Tags.vi"("Name Values"=w523, "Group Names"=w524, "Notes"="Notes") -> ("Name Value Group"=w514:string[][])  [unwired: 12 in]
        n242 = Array Size(array=w514) -> (size(s)=w521:i32[])
        n243 = Index Array(array=w521, index=0) -> (element=w519:i32)
        n244 = Transpose 2D Array(2D array=w514) -> (transposed array=w517:string[][])
        n245 = Initialize Array("Sample", w519) -> (w516:string[])
        n246 = Build Array (concatenate)(w517, w516) -> (w515:string[][])
        n247 = call "Name Value Write Tags.vi"("File Path"=w529, "Tags Group Array"=w514) -> ()  [unwired: 13 in, 1 out]
        n248 = Transpose 2D Array(2D array=w515) -> (transposed array=w510:string[][])
        n249 = call "Name Value Sort for New.vi"("Organized Name Values"=w510) -> ("Sorted"=w511:string[][])  [unwired: 14 in]
        n250 = for {
          tunnel: w513 -> [w540] mode=indexing
          tunnel: w512 -> [w539] mode=indexing
          tunnel: w511 -> [w536]
          i -> [w535]
          n251 = Unbundle By Name(w539) -> ("Sorted Tags"=w533:string[], "First Letters"=w538:string[], "Letter Indices"=w537:i32[])
          n252 = Index Array(array=w536, index (col)=w535) -> (element=w534:string[])  [unwired: 1 in]
          n253 = call "Name Value Check New.vi"("Tags"=w534, "Sorted Tags"=w533, "First Letters"=w538, "Letter Indicies"=w537) -> ("New Tags"=w541:string[], "New Tags Bool"=w542:bool)  [unwired: 10 in]
          n254 = case shown="True" w542 {
            tunnel: w541 -> [_ w546]
            tunnel: w540 -> [_ w544]
            tunnel: w533 -> [_ w543]
            frame False {
            }
            frame True {
              n255 = Build Array (concatenate)(w543, w546) -> (w545:string[])
              n256 = Write to Text File(file (use dialog)=w544, text=w545) -> ()  [unwired: 2 in, 3 out]
            }
          }
        }
        n257 = Not A Number/Path/Refnum?(number/path/refnum="Save Path") -> (NaN/Path/Refnum?=w528:bool)
        n258 = Empty String/Path?(string/path="Save Path") -> (empty?=w527:bool)
        n259 = Or(x=w528, y=w527) -> (x .or. y?=w525:bool)
        n260 = case shown="False" w525 {
          tunnel: "Save Path" -> [w548 _]
          tunnel: w510 -> [w547 _]
          frame False {
            n261 = call "Name Value Write Data.vi"("Save Path"=w548, "NameValues"=w547) -> ()  [unwired: 14 in]
          }
          frame True {
          }
        }
      }
      event "Cancel": Value Change {
        n262 = event-data() -> ()  [unwired: 1 in, 3 out]
      }
    }
  }
  n263 = Unbundle By Name(w66) -> ("Left"=w68:i16, "Top"=w53:i16)
  n264 = Add(x=w53, y=w51) -> (x+y=w52:i16)
  n265 = Add(x=w68, y=w70) -> (x+y=w54:i16)
  n266 = Bundle By Name(cluster=w66, "Right"=w54, "Bottom"=w52) -> (w67:T6)
  n267 = property class="VI"(reference=w65, "Front Panel.PanelBounds"=w67) -> (reference out=w11:refnum<vi>)  [unwired: 1 in, 1 out]
  n268 = invoke class="VI" method="FP.Center"(reference=w11) -> (reference out=w13:refnum<vi>)  [unwired: 2 in, 2 out]
  n269 = Close Reference(reference=w13) -> ()  [unwired: 1 in, 1 out]
  n270 = local write "Save"(w1) -> ()
